vi "Autonomous Independent.vi"   [LabVIEW 2019]
doc: "This VI is called when autonomous begins, and will automatically be terminated when autonomous ends. You can carry out timed or sensor driven robot movement independently without needing to return to the caller."
uses:
  <vilib>/Rock Robotics/WPI/ThirdParty/Phoenix-LabVIEW/Motor Controller/Controls/CTRE_Phoenix_MotorControl_ControlMode.ctl
  <vilib>/Rock Robotics/WPI/Solenoid/WPI_SolenoidValue.ctl
  <vilib>/Rock Robotics/Network Tables/NT Read String.vi
  <vilib>/Rock Robotics/WPI/Utilities/WPI_GetSetVariantRefNum.vi
  <vilib>/Rock Robotics/Network Tables/NT Write Number.vi
  <vilib>/Rock Robotics/WPI/Solenoid/WPI_SolenoidSetEnum.vi
  <vilib>/Rock Robotics/Network Tables/NT Read Number.vi
  <vilib>/addons/control/pid/pid.llb/PID (DBL).vi
  <vilib>/addons/control/pid/NI_PID_pid.lvlib
  <vilib>/Rock Robotics/Network Tables/NT Write Numeric Array.vi
panel:
  # "Be sure to right-click and choose Data Operations>>Make Current Value default if you want to save the array values with the VI"
types:
  T1 = typedef "WPI_JoystickDevRef.ctl" = cluster{"Device":T2}
  T2 = typedef "WPI_JoystickDeviceEnum.ctl" = enum16{"USB 0", "USB 1", "USB 2", "USB 3", "USB 4", "USB 5"}
  T3 = typedef "WPI_MotorControlDeviceRef.ctl" = cluster{"DeviceStatus":errorcluster, "Type":T4, "PWM":cluster{"PWM Channel":T5, "DeadBand":T6}, "CAN":cluster{"Device Number":u8, "SetOutput VI Ref":variant, "GetOutput VI Ref":variant, "Enable VI Ref":variant, "Disable VI Ref":variant, "Data":variant}, "Invert":bool, "DIO PWM":cluster{"PWM \"Enable\" Channel":T5, "DIOChannel":T7, "PWM Rate":dbl}}
  T4 = typedef "WPI_MotorControlType.ctl" = enum16{"PWM", "CAN", "DIO PWM"}
  T5 = typedef "FPGA_DIOPWMChannel.ctl" = enum8{"PWM 0", "PWM 1", "PWM 2", "PWM 3", "PWM 4", "PWM 5", "PWM 6", "PWM 7", "PWM 8", "PWM 9", "PWM MXP 0", "PWM MXP 1", "PWM MXP 2", "PWM MXP 3", "PWM MXP 4", "PWM MXP 5", "PWM MXP 6", "PWM MXP 7", "PWM MXP 8", "PWM MXP 9", "Invalid"}
  T6 = typedef "WPI_PWMDeadband.ctl" = cluster{"Name":string, "maxPositivePwm":i32, "minPositivePwm":i32, "centerPwm":i32, "maxNegativePwm":i32, "minNegativePwm":i32, "angularRange":u16}
  T7 = typedef "FPGA_DIOChannel.ctl" = enum8{"DIO 0", "DIO 1", "DIO 2", "DIO 3", "DIO 4", "DIO 5", "DIO 6", "DIO 7", "DIO 8", "DIO 9", "DIO MXP 0", "DIO MXP 1", "DIO MXP 2", "DIO MXP 3", "DIO MXP 4", "DIO MXP 5", "DIO MXP 6", "DIO MXP 7", "DIO MXP 8", "DIO MXP 9", "DIO MXP 10", "DIO MXP 11", "DIO MXP 12", "DIO MXP 13", "DIO MXP 14", "DIO MXP 15", "SPI Port CS1", "SPI Port CS2", "SPI Port CS3", "SPI Port MISO", "SPI Port MOSI", "Invalid"}
  T8 = typedef "WPI_RobotDriveDevRef.ctl" = cluster{"DevStatus":errorcluster, "Motors[]":T3[], "Square Inputs":bool, "Max Output":dbl}
  T9 = typedef "WPI_GyroDevRef.ctl" = cluster{"DevStatus":errorcluster, "Analog Channel":T10, "Gain (VoltsPerDegree/Second)":dbl, "Gyro Type":enum16{"Analog", "XRS450"}, "Handle":i32, "SPI Bus":T11, "Device Found":bool, "Sample Rate":dbl, "Calibrate On Open":bool, "Offset":dbl}
  T10 = typedef "FPGA_AIChannel.ctl" = enum8{"AI 0", "AI 1", "AI 2", "AI 3", "AI MXP 0", "AI MXP 1", "AI MXP 2", "AI MXP 3", "Invalid"}
  T11 = typedef "spi_bus.ctl" = enum16{"SPI On-Board, CS0", "SPI On-Board, CS1", "SPI On-Board, CS2", "SPI On-Board, CS3", "SPI MXP", "Invalid"}
  T12 = typedef "WPI_SolenoidDevRef.ctl" = cluster{"DevStatus":errorcluster, "Pneumatics Control Module":u8, "Forward Solenoid Channel":T13, "Reverse Solenoid Channel":T13}
  T13 = typedef "WPI_SolenoidChannel.ctl" = enum8{"Solenoid 0", "Solenoid 1", "Solenoid 2", "Solenoid 3", "Solenoid 4", "Solenoid 5", "Solenoid 6", "Solenoid 7", "Invalid"}
  T14 = typedef "WPI_SolenoidValue.ctl" = enum16{"Off", "On", "Forward", "Reverse"}
  T15 = cluster{"proportional gain (Kc)":dbl, "integral time (Ti, min)":dbl, "derivative time (Td, min)":dbl}
  T16 = typedef "CTRE_Phoenix_MotorControl_ControlMode.ctl" = u16
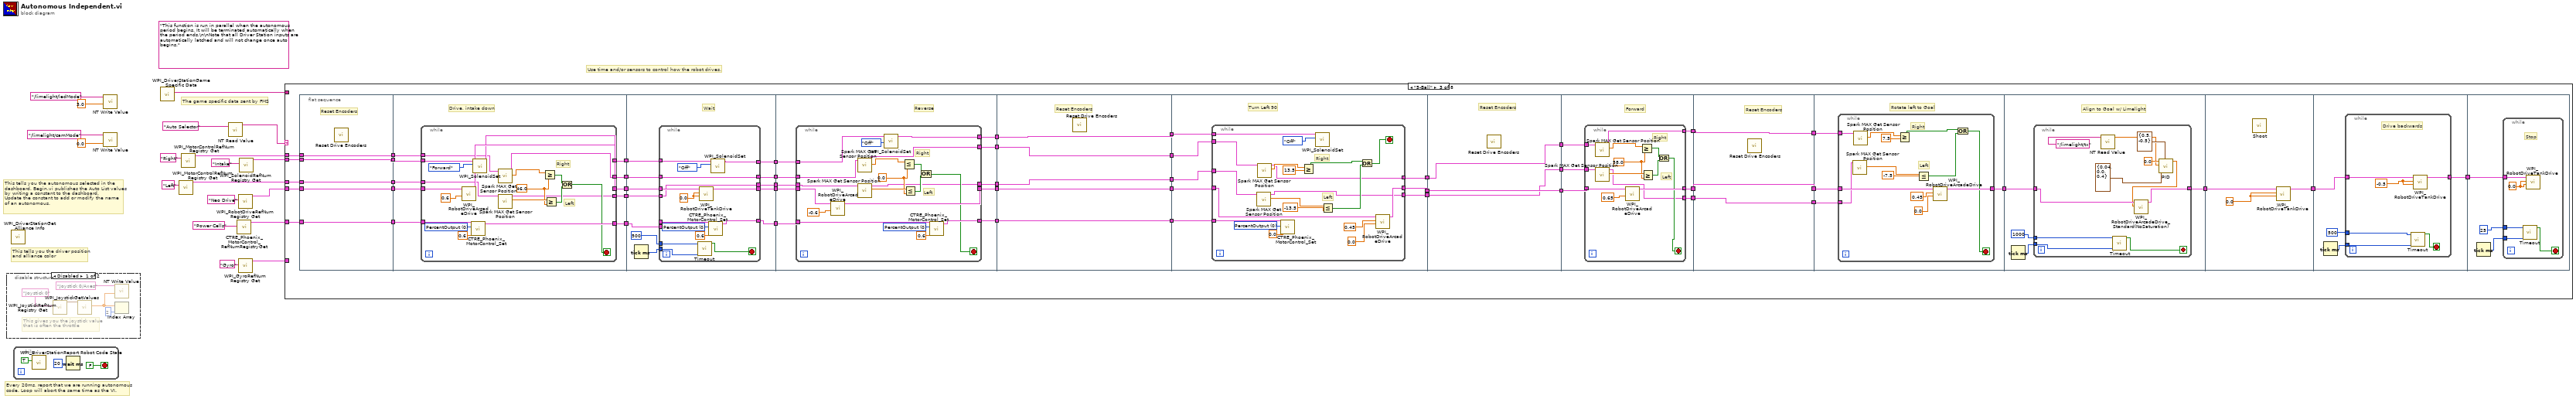
[diagram p0: block diagram]
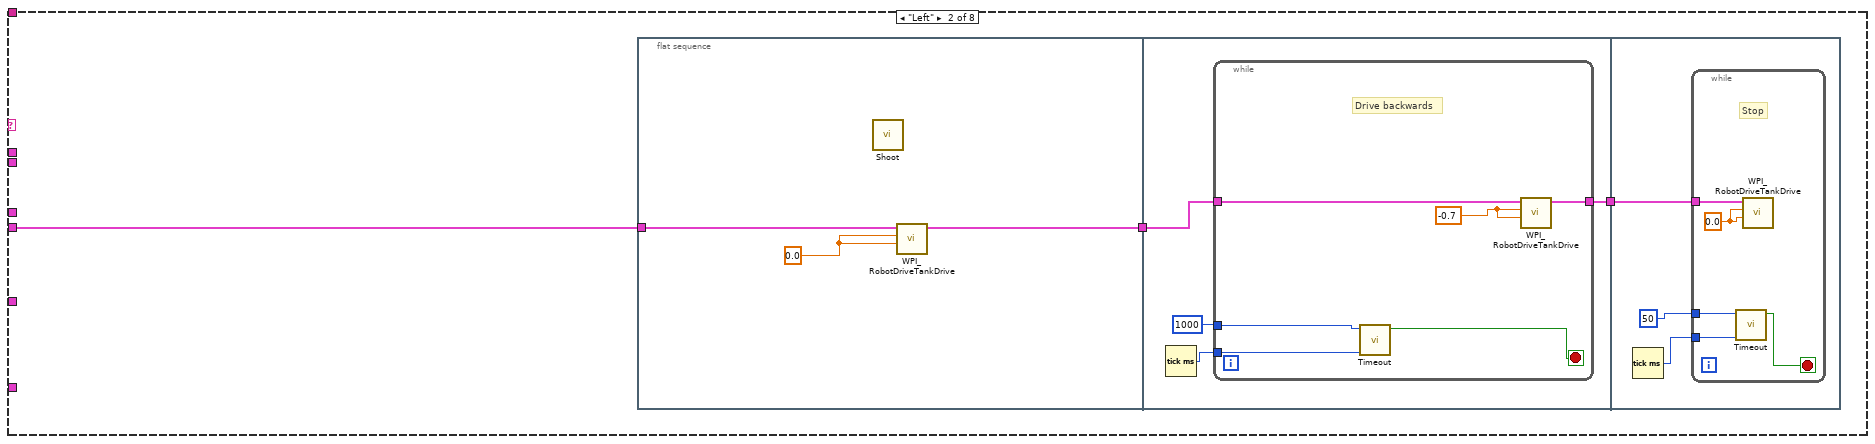
[diagram p4: hidden frame]
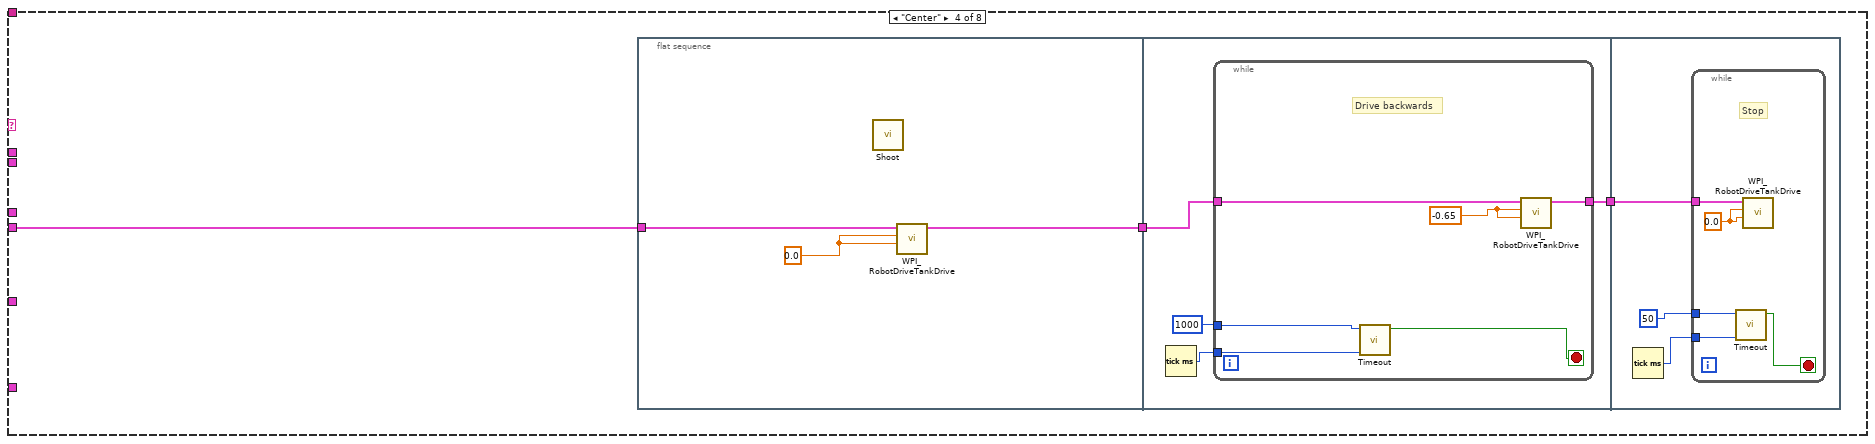
[diagram p5: hidden frame]
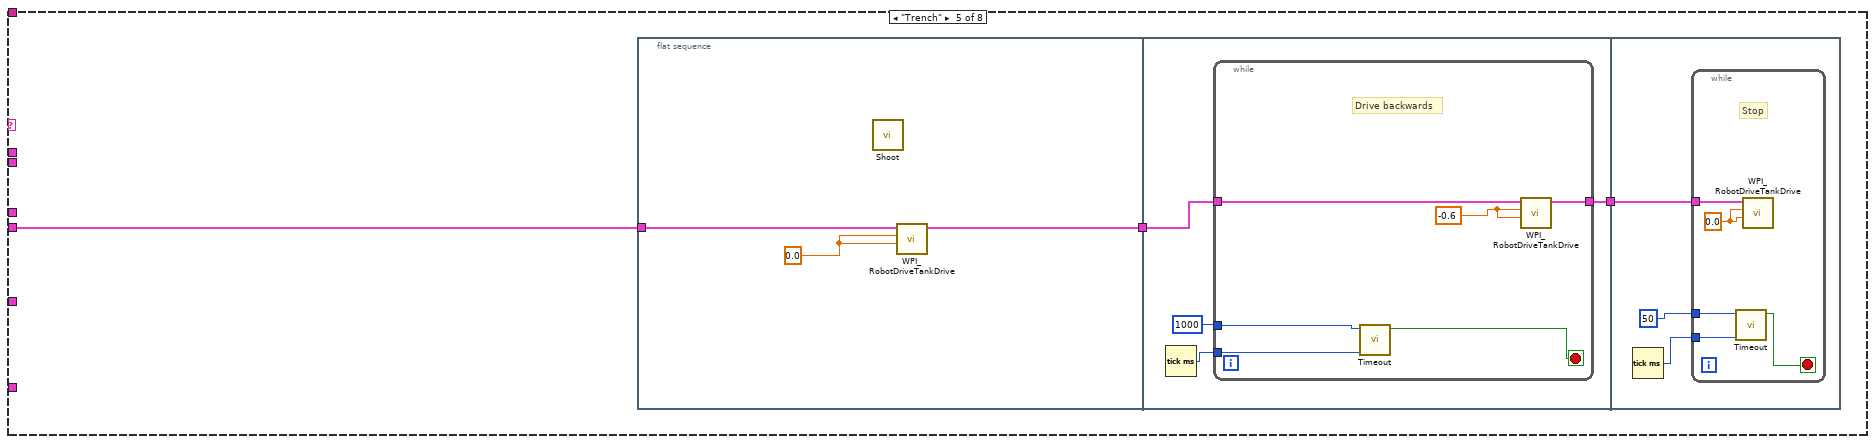
[diagram p6: hidden frame]
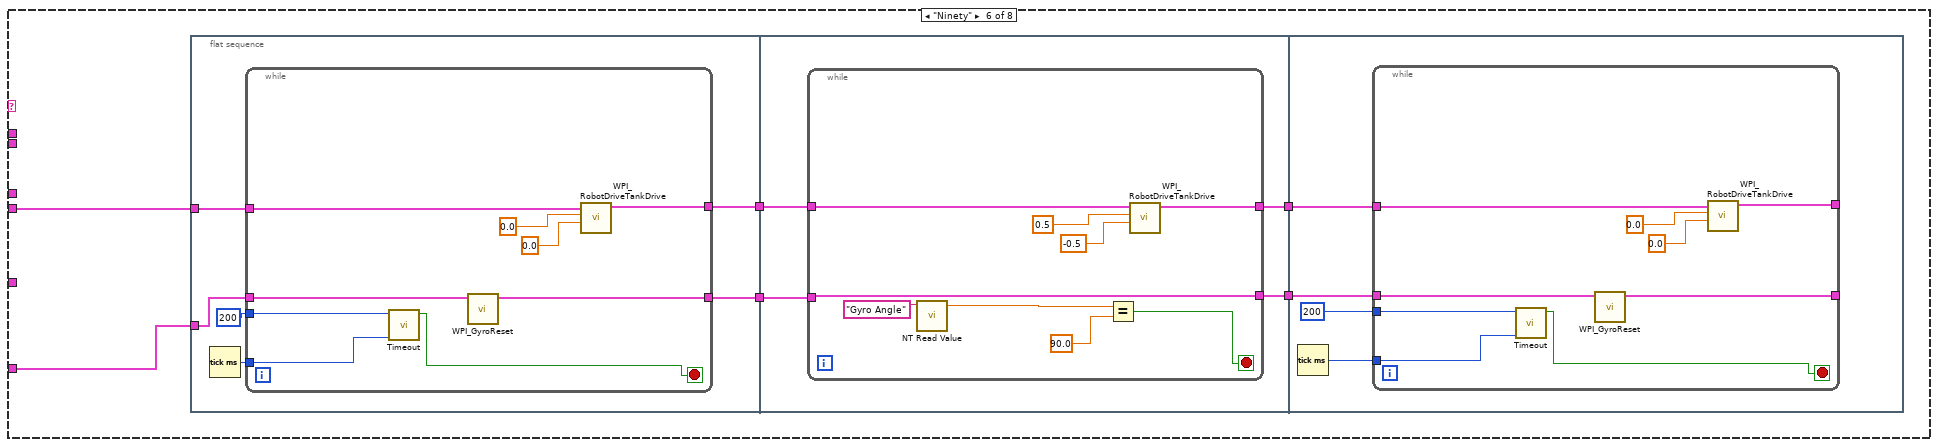
[diagram p7: hidden frame]
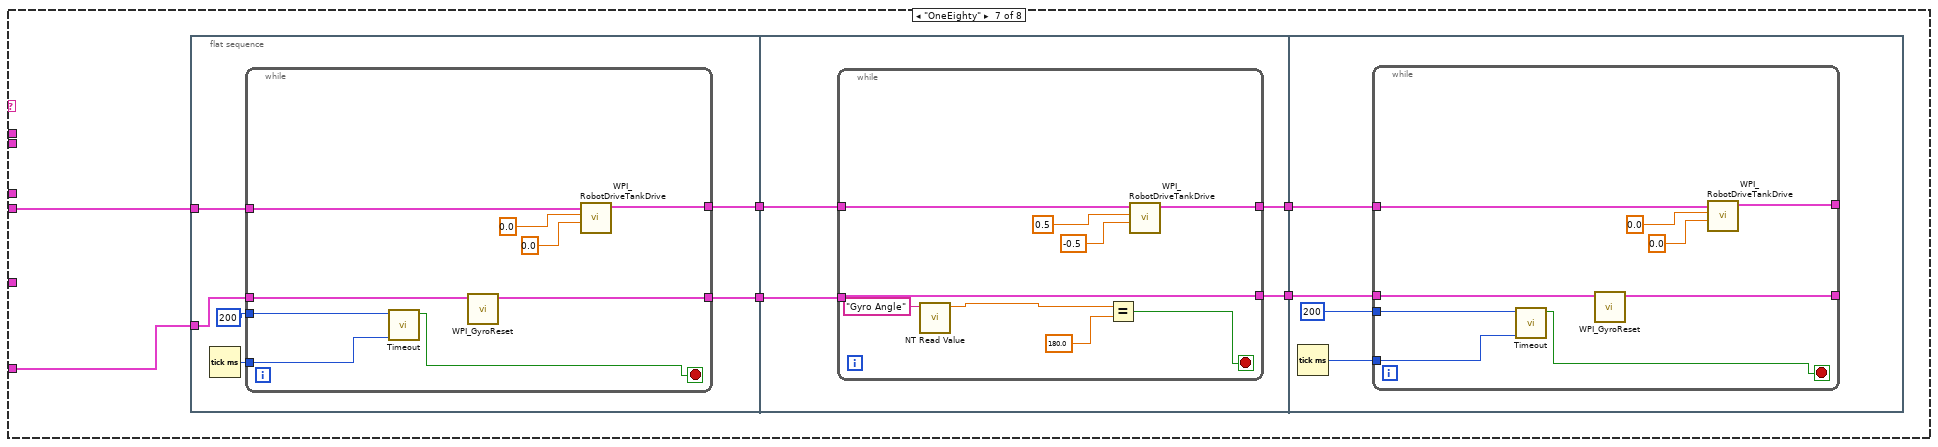
[diagram p8: hidden frame]
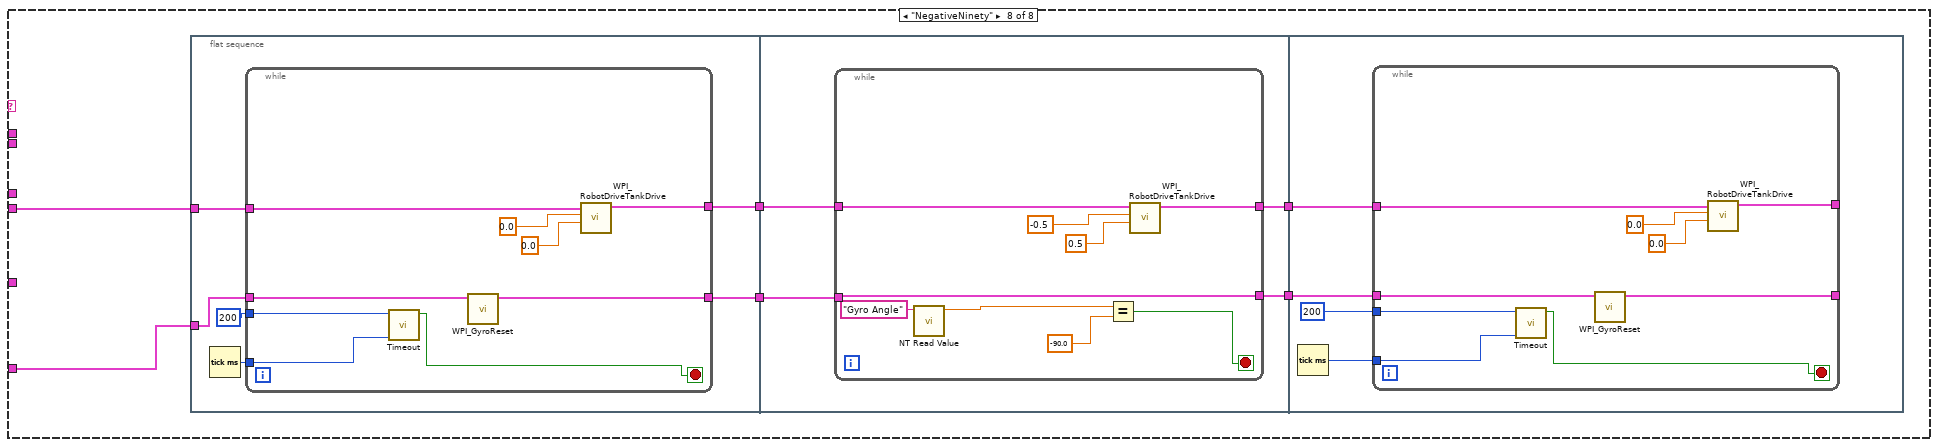
[diagram p9: hidden frame]
diagram:
  (unwired) "This function is run in parallel when the autonomous period begins. It will be terminated automatically when the period ends.\n\nNote that all Driver Station inputs are automatically latched and will not change once auto begins."
  # "The game specific data sent by FMS"
  # "This tells you the autonomous selected in the \ndashboard. Begin.vi publishes the Auto List values\nby writing a constant to the dashboard.\nUpdate the constant to add or modify the name\nof an autonomous."
  # "Every 20ms, report that we are running autonomous\ncode. Loop will abort the same time as the VI."
  # "Use time and/or sensors to control how the robot drives."
  # "This tells you the driver position\nand alliance color"
  n1 = disable-structure shown="Disabled" {
    frame Disabled {
      # "This gives you the joystick value\nthat is often the throttle"
      n2 = call <vilib>:"WPI_JoystickRefNum Registry Get.vi"("refnum name"="Joystick 0") -> ("JoystickDevRef"=w23:T1)  [unwired: 1 in, 9 out]
      n3 = call <vilib>:"WPI_JoystickGetValues.vi"("JoystickDevRef"=w23) -> ("Axes"=w21:dbl[])  [unwired: 6 in, 4 out]
      n4 = call-poly <vilib>:"NT Write Value.vi"("Numeric Array"=w21, "Name"="Joystick 0/Axes") -> ()  [unwired: 9 in, 1 out]
      n5 = Index Array(array=w21, index=2) -> ()  [unwired: 1 out]
    }
    frame Enabled {
    }
  }
  n6 = call <vilib>:"WPI_DriverStationGet Alliance Info.vi"() -> ()  [unwired: 12 out]
  n7 = while {
    stop <- FALSE stop-if-true
    n8 = call <vilib>:"WPI_DriverStationReport Robot Code State.vi"("Autonomous"=TRUE) -> ()  [unwired: 10 in, 1 out]
    n9 = Wait (ms)(milliseconds to wait=u32 20) -> ()  [unwired: 1 out]
  }
  n10 = call-poly <vilib>:"NT Write Value.vi"("Numeric"=3.0, "Name"="/limelight/ledMode") -> ()  [unwired: 9 in, 1 out]
  n11 = call-poly <vilib>:"NT Write Value.vi"("Numeric"=0.0, "Name"="/limelight/camMode") -> ()  [unwired: 9 in, 1 out]
  n12 = call <vilib>:"WPI_DriverStationGame Specific Data.vi"() -> ("Game Specific Data"=w18:string)  [unwired: 11 in]
  n13 = call <vilib>:"WPI_MotorControlRefNum Registry Get.vi"("refnum name"="Left") -> ("MotorControlDevRef"=w5:T3)  [unwired: 9 in, 1 out]
  n14 = call <vilib>:"WPI_MotorControlRefNum Registry Get.vi"("refnum name"="Right") -> ("MotorControlDevRef"=w4:T3)  [unwired: 9 in, 1 out]
  n15 = call-poly <vilib>:"NT Read Value.vi"("Name"="Auto Selector") -> ("String"=w3:string)  [unwired: 9 in, 1 out]
  n16 = call <vilib>:"CTRE_Phoenix_MotorControl_RefNumRegistryGet.vi"("refnum name"="Power Cells") -> ("PhoenixMotorControlDevRef"=w12:T3)  [unwired: 9 in, 1 out]
  n17 = call <vilib>:"WPI_RobotDriveRefNum Registry Get.vi"("refnum name"="Neo Drive") -> ("RobotDriveDevRef"=w16:T8)  [unwired: 9 in, 1 out]
  n18 = call <vilib>:"WPI_GyroRefNum Registry Get.vi"("refnum name"="Gyro") -> ("GyroDevRef"=w1:T9)  [unwired: 9 in, 1 out]
  n19 = call <vilib>:"WPI_SolenoidRefNum Registry Get.vi"("refnum name"="Intake") -> ("SolenoidDevRef"=w13:T12)  [unwired: 9 in, 1 out]
  n20 = case shown="\"5-Ball\"" w3 {
    tunnel: w18 -> [_ _ _ _ _ _ _ _]
    tunnel: w16 -> [_ w30 w97 w303 w327 w354 w401 w448]
    tunnel: w13 -> [_ _ w94 _ _ _ _ _]
    tunnel: w12 -> [_ _ w93 _ _ _ _ _]
    tunnel: w5 -> [_ _ w78 _ _ _ _ _]
    tunnel: w4 -> [_ _ w79 _ _ _ _ _]
    tunnel: w1 -> [_ _ _ _ _ w353 w400 w447]
    frame Default {
      # "You can put your main auto here, or you can right-click on the case and make any\nother frame be the default case."
      # "This is the frame that will execute if no selection is made, or if it is not recognized"
    }
    frame "Left" {
      n21 = flat-sequence {
        tunnel: w30 -> [w33]
        tunnel: [w32] -> w29
        tunnel: w29 -> [w35]
        tunnel: [w34] -> w28
        tunnel: w28 -> [w44]
        frame #0 {
          w31 = 0.0 ("Left axis value")
          n22 = call "Shoot.vi"() -> ()  [unwired: 12 in]
          n23 = call <vilib>:"WPI_RobotDriveTankDrive.vi"("Right axis value"=w31, "Left axis value"=w31, "RobotDriveDevRef"=w33) -> ("RobotDriveDevRef"=w32:T8)  [unwired: 6 in, 2 out]
        }
        frame #1 {
          n24 = Tick Count (ms)() -> (millisecond timer value=w37:u32)
          n25 = while {
            tunnel: w35 -> [w43]
            tunnel: w37 -> [w41]
            tunnel: 1000 -> [w40]
            tunnel: [w38] -> w34
            stop <- w39 stop-if-true
            w42 = -0.7 ("Left axis value")
            # "Drive backwards"
            n26 = call "Timeout.vi"("Start Time In"=w41, "Limit In"=w40) -> ("Timeout"=w39:bool)  [unwired: 8 in, 1 out]
            n27 = call <vilib>:"WPI_RobotDriveTankDrive.vi"("Right axis value"=w42, "Left axis value"=w42, "RobotDriveDevRef"=w43) -> ("RobotDriveDevRef"=w38:T8)  [unwired: 6 in, 2 out]
          }
        }
        frame #2 {
          n28 = Tick Count (ms)() -> (millisecond timer value=w46:u32)
          n29 = while {
            tunnel: w46 -> [w51]
            tunnel: 50 -> [w50]
            tunnel: w44 -> [w48]
            stop <- w49 stop-if-true
            w47 = 0.0 ("Left axis value")
            # "Stop"
            n30 = call "Timeout.vi"("Start Time In"=w51, "Limit In"=w50) -> ("Timeout"=w49:bool)  [unwired: 8 in, 1 out]
            n31 = call <vilib>:"WPI_RobotDriveTankDrive.vi"("Right axis value"=w47, "Left axis value"=w47, "RobotDriveDevRef"=w48) -> ()  [unwired: 6 in, 3 out]
          }
        }
      }
    }
    frame "5-Ball" {
      n32 = flat-sequence {
        tunnel: w78 -> [w100]
        tunnel: w79 -> [w98]
        tunnel: w93 -> [w102]
        tunnel: w94 -> [w99]
        tunnel: w97 -> [w101]
        tunnel: [w102] -> w71
        tunnel: [w101] -> w58
        tunnel: [w100] -> w57
        tunnel: [w99] -> w56
        tunnel: [w98] -> w55
        tunnel: [w110] -> w90
        tunnel: [w108] -> w88
        tunnel: [w107] -> w87
        tunnel: [w104] -> w77
        tunnel: [w103] -> w76
        tunnel: w71 -> [w112]
        tunnel: w58 -> [w111]
        tunnel: w57 -> [w105]
        tunnel: w56 -> [w109]
        tunnel: w55 -> [w106]
        tunnel: w90 -> [w140]
        tunnel: [w143] -> w89
        tunnel: w88 -> [w144]
        tunnel: w87 -> [w142]
        tunnel: [w141] -> w86
        tunnel: [w137] -> w81
        tunnel: w77 -> [w136]
        tunnel: w76 -> [w135]
        tunnel: [w134] -> w75
        tunnel: [w133] -> w74
        tunnel: [w168] -> w85
        tunnel: w89 -> [w169]
        tunnel: w86 -> [w167]
        tunnel: [w166] -> w83
        tunnel: w81 -> [w165]
        tunnel: [w164] -> w80
        tunnel: w75 -> [w163]
        tunnel: w74 -> [w162]
        tunnel: [w161] -> w73
        tunnel: [w160] -> w72
        tunnel: w85 -> [w194]
        tunnel: [w194] -> w84
        tunnel: w83 -> [w193]
        tunnel: [w193] -> w82
        tunnel: w80 -> [w190]
        tunnel: w73 -> [w191]
        tunnel: w72 -> [w192]
        tunnel: [w192] -> w54
        tunnel: [w191] -> w53
        tunnel: [w190] -> w52
        tunnel: w84 -> [w202]
        tunnel: [w201] -> w70
        tunnel: w82 -> [w200]
        tunnel: [w196] -> w68
        tunnel: [w195] -> w67
        tunnel: w54 -> [w199]
        tunnel: w53 -> [w198]
        tunnel: w52 -> [w197]
        tunnel: w70 -> [w225]
        tunnel: [w225] -> w69
        tunnel: w68 -> [w224]
        tunnel: w67 -> [w223]
        tunnel: [w224] -> w66
        tunnel: [w223] -> w65
        tunnel: w69 -> [w231]
        tunnel: [w230] -> w64
        tunnel: w66 -> [w229]
        tunnel: w65 -> [w228]
        tunnel: [w227] -> w62
        tunnel: [w226] -> w61
        tunnel: w64 -> [w247]
        tunnel: [w247] -> w63
        tunnel: w62 -> [w246]
        tunnel: w61 -> [w245]
        tunnel: [w246] -> w60
        tunnel: [w245] -> w59
        tunnel: w63 -> [w251]
        tunnel: [w250] -> w92
        tunnel: w60 -> [w249]
        tunnel: w59 -> [w248]
        tunnel: w92 -> [w268]
        tunnel: [w267] -> w91
        tunnel: [w281] -> w96
        tunnel: w91 -> [w282]
        tunnel: w96 -> [w284]
        tunnel: [w283] -> w95
        tunnel: w95 -> [w293]
        frame #0 {
          # "Reset Encoders"
          n33 = call "Reset Drive Encoders.vi"() -> ()  [unwired: 12 in]
        }
        frame #1 {
          # "Drive, intake down"
          n34 = while {
            tunnel: w112 -> [w132]
            tunnel: w111 -> [w129]
            tunnel: [w128] -> w110
            tunnel: w109 -> [w126]
            tunnel: [w124] -> w108
            tunnel: [w123] -> w107
            tunnel: w106 -> [w116]
            tunnel: w105 -> [w115]
            tunnel: [w114] -> w104
            tunnel: [w113] -> w103
            stop <- w117 stop-if-true
            w120 = 46.0 ("y")
            w131 = T16 0 items=["PercentOutput"=0, "Position"=1, "Velocity"=2, "Current"=3, "Follower"=5, "MotionProfile"=6, "MotionMagic"=7, "MotionProfileArc"=10, "Disabled"=15] ("Control Mode")
            # "Left"
            # "Right"
            n35 = call-poly <vilib>:"WPI_RobotDriveArcadeDrive.vi"("Y axis value"=0.6 ("Left axis value"), "RobotDriveDevRef"=w129) -> ("RobotDriveDevRef"=w128:T8)  [unwired: 7 in, 2 out]
            n36 = call <vilib>:"CTRE_Phoenix_MotorControl_Set.vi"("Output"=0.6, "Control Mode"=w131, "PhoenixMotorControlDevRef"=w132) -> ("PhoenixMotorControlDevRef"=w123:T3)  [unwired: 7 in, 1 out]
            n37 = call-poly <vilib>:"WPI_SolenoidSet.vi"("Value"=WPI_SolenoidValue."Forward", "SolenoidDevRef"=w126) -> ("SolenoidDevRef"=w124:T12)  [unwired: 8 in, 1 out]
            n38 = call <vilib>:"Spark MAX Get Sensor Position.vi"("MotorControlDevRef in"=w116) -> ("Sensor Position"=w122:dbl, "MotorControlDevRef out"=w114:T3)  [unwired: 7 in, 2 out]
            n39 = call <vilib>:"Spark MAX Get Sensor Position.vi"("MotorControlDevRef in"=w115) -> ("Sensor Position"=w121:dbl, "MotorControlDevRef out"=w113:T3)  [unwired: 7 in, 2 out]
            n40 = Greater Or Equal?(x=w122, y=w120) -> (x >= y?=w118:bool)
            n41 = Greater Or Equal?(x=w121, y=w120) -> (x >= y?=w119:bool)
            n42 = Or(x=w118, y=w119) -> (x .or. y?=w117:bool)
          }
        }
        frame #2 {
          # "Wait"
          n43 = Tick Count (ms)() -> (millisecond timer value=w139:u32)
          n44 = while {
            tunnel: [w148] -> _
            tunnel: 500 -> [w156]
            tunnel: w139 -> [w155]
            tunnel: w140 -> [w154]
            tunnel: [w153] -> w143
            tunnel: w144 -> [w151]
            tunnel: [w149] -> w141
            tunnel: w142 -> [w148]
            tunnel: [w147] -> w137
            tunnel: w136 -> [w146]
            tunnel: w135 -> [w145]
            tunnel: [w146] -> w134
            tunnel: [w145] -> w133
            stop <- w157 stop-if-true
            w152 = 0.0 ("Left axis value")
            w159 = T16 0 items=["PercentOutput"=0, "Position"=1, "Velocity"=2, "Current"=3, "Follower"=5, "MotionProfile"=6, "MotionMagic"=7, "MotionProfileArc"=10, "Disabled"=15] ("Control Mode")
            n45 = call "Timeout.vi"("Start Time In"=w155, "Limit In"=w156) -> ("Timeout"=w157:bool)  [unwired: 8 in, 1 out]
            n46 = call <vilib>:"WPI_RobotDriveTankDrive.vi"("Right axis value"=w152, "Left axis value"=w152, "RobotDriveDevRef"=w154) -> ("RobotDriveDevRef"=w153:T8)  [unwired: 6 in, 2 out]
            n47 = call <vilib>:"CTRE_Phoenix_MotorControl_Set.vi"("Output"=0.6, "Control Mode"=w159, "PhoenixMotorControlDevRef"=w148) -> ("PhoenixMotorControlDevRef"=w149:T3)  [unwired: 7 in, 1 out]
            n48 = call-poly <vilib>:"WPI_SolenoidSet.vi"("Value"=WPI_SolenoidValue."Off", "SolenoidDevRef"=w151) -> ("SolenoidDevRef"=w147:T12)  [unwired: 8 in, 1 out]
          }
        }
        frame #3 {
          # "Reverse"
          n49 = while {
            tunnel: w167 -> [w189]
            tunnel: w169 -> [w186]
            tunnel: [w185] -> w168
            tunnel: [w183] -> w166
            tunnel: w165 -> [w181]
            tunnel: [w180] -> w164
            tunnel: w163 -> [w174]
            tunnel: w162 -> [w173]
            tunnel: [w171] -> w161
            tunnel: [w170] -> w160
            stop <- w172 stop-if-true
            w177 = 0.0 ("y")
            w188 = T16 0 items=["PercentOutput"=0, "Position"=1, "Velocity"=2, "Current"=3, "Follower"=5, "MotionProfile"=6, "MotionMagic"=7, "MotionProfileArc"=10, "Disabled"=15] ("Control Mode")
            # "Left"
            # "Right"
            n50 = call-poly <vilib>:"WPI_RobotDriveArcadeDrive.vi"("Y axis value"=-0.6 ("Left axis value"), "RobotDriveDevRef"=w186) -> ("RobotDriveDevRef"=w185:T8)  [unwired: 7 in, 2 out]
            n51 = call <vilib>:"Spark MAX Get Sensor Position.vi"("MotorControlDevRef in"=w174) -> ("Sensor Position"=w179:dbl, "MotorControlDevRef out"=w171:T3)  [unwired: 7 in, 2 out]
            n52 = call <vilib>:"Spark MAX Get Sensor Position.vi"("MotorControlDevRef in"=w173) -> ("Sensor Position"=w178:dbl, "MotorControlDevRef out"=w170:T3)  [unwired: 7 in, 2 out]
            n53 = call-poly <vilib>:"WPI_SolenoidSet.vi"("Value"=WPI_SolenoidValue."Off", "SolenoidDevRef"=w181) -> ("SolenoidDevRef"=w180:T12)  [unwired: 8 in, 1 out]
            n54 = Less Or Equal?(x=w179, y=w177) -> (x <= y?=w175:bool)
            n55 = Less Or Equal?(x=w178, y=w177) -> (x <= y?=w176:bool)
            n56 = Or(x=w175, y=w176) -> (x .or. y?=w172:bool)
            n57 = call <vilib>:"CTRE_Phoenix_MotorControl_Set.vi"("Output"=0.6, "Control Mode"=w188, "PhoenixMotorControlDevRef"=w189) -> ("PhoenixMotorControlDevRef"=w183:T3)  [unwired: 7 in, 1 out]
          }
        }
        frame #4 {
          # "Reset Encoders"
          n58 = call "Reset Drive Encoders.vi"() -> ()  [unwired: 12 in]
        }
        frame #5 {
          # "Turn Left 90"
          n59 = while {
            tunnel: w202 -> [w222]
            tunnel: [w221] -> w201
            tunnel: w200 -> [w216]
            tunnel: w198 -> [w215]
            tunnel: w199 -> [w214]
            tunnel: w197 -> [w205]
            tunnel: [w204] -> w196
            tunnel: [w203] -> w195
            stop <- w213 stop-if-true
            w218 = T16 0 items=["PercentOutput"=0, "Position"=1, "Velocity"=2, "Current"=3, "Follower"=5, "MotionProfile"=6, "MotionMagic"=7, "MotionProfileArc"=10, "Disabled"=15] ("Control Mode")
            # "Left"
            # "Right"
            n60 = call <vilib>:"Spark MAX Get Sensor Position.vi"("MotorControlDevRef in"=w214) -> ("Sensor Position"=w208:dbl, "MotorControlDevRef out"=w203:T3)  [unwired: 7 in, 2 out]
            n61 = call <vilib>:"Spark MAX Get Sensor Position.vi"("MotorControlDevRef in"=w215) -> ("Sensor Position"=w212:dbl, "MotorControlDevRef out"=w204:T3)  [unwired: 7 in, 2 out]
            n62 = call <vilib>:"CTRE_Phoenix_MotorControl_Set.vi"("Output"=0.0, "Control Mode"=w218, "PhoenixMotorControlDevRef"=w216) -> ()  [unwired: 7 in, 2 out]
            n63 = Greater Or Equal?(x=w212, y=13.5) -> (x >= y?=w210:bool)
            n64 = call-poly <vilib>:"WPI_SolenoidSet.vi"("Value"=WPI_SolenoidValue."Off", "SolenoidDevRef"=w205) -> ()  [unwired: 8 in, 2 out]
            n65 = Less Or Equal?(x=w208, y=-13.5) -> (x <= y?=w207:bool)
            n66 = Or(x=w210, y=w207) -> (x .or. y?=w213:bool)
            n67 = call-poly <vilib>:"WPI_RobotDriveArcadeDrive.vi"("Y axis value"=0.0 ("Left axis value"), "X axis value"=0.45 ("Left axis value"), "RobotDriveDevRef"=w222) -> ("RobotDriveDevRef"=w221:T8)  [unwired: 6 in, 2 out]
          }
        }
        frame #6 {
          # "Reset Encoders"
          n68 = call "Reset Drive Encoders.vi"() -> ()  [unwired: 12 in]
        }
        frame #7 {
          # "Forward"
          n69 = while {
            tunnel: w231 -> [w244]
            tunnel: [w243] -> w230
            tunnel: w229 -> [w235]
            tunnel: w228 -> [w234]
            tunnel: [w233] -> w227
            tunnel: [w232] -> w226
            stop <- w236 stop-if-true
            w239 = 58.0 ("y")
            # "Left"
            # "Right"
            n70 = call <vilib>:"Spark MAX Get Sensor Position.vi"("MotorControlDevRef in"=w235) -> ("Sensor Position"=w241:dbl, "MotorControlDevRef out"=w233:T3)  [unwired: 7 in, 2 out]
            n71 = call <vilib>:"Spark MAX Get Sensor Position.vi"("MotorControlDevRef in"=w234) -> ("Sensor Position"=w240:dbl, "MotorControlDevRef out"=w232:T3)  [unwired: 7 in, 2 out]
            n72 = call-poly <vilib>:"WPI_RobotDriveArcadeDrive.vi"("Y axis value"=0.65 ("Left axis value"), "RobotDriveDevRef"=w244) -> ("RobotDriveDevRef"=w243:T8)  [unwired: 7 in, 2 out]
            n73 = Greater Or Equal?(x=w241, y=w239) -> (x >= y?=w237:bool)
            n74 = Greater Or Equal?(x=w240, y=w239) -> (x >= y?=w238:bool)
            n75 = Or(x=w237, y=w238) -> (x .or. y?=w236:bool)
          }
        }
        frame #8 {
          # "Reset Encoders"
          n76 = call "Reset Drive Encoders.vi"() -> ()  [unwired: 12 in]
        }
        frame #9 {
          # "Rotate left to Goal"
          n77 = while {
            tunnel: w251 -> [w264]
            tunnel: [w263] -> w250
            tunnel: w249 -> [w253]
            tunnel: w248 -> [w252]
            stop <- w254 stop-if-true
            # "Left"
            # "Right"
            n78 = call <vilib>:"Spark MAX Get Sensor Position.vi"("MotorControlDevRef in"=w252) -> ("Sensor Position"=w256:dbl)  [unwired: 7 in, 3 out]
            n79 = call <vilib>:"Spark MAX Get Sensor Position.vi"("MotorControlDevRef in"=w253) -> ("Sensor Position"=w260:dbl)  [unwired: 7 in, 3 out]
            n80 = Greater Or Equal?(x=w260, y=7.5) -> (x >= y?=w258:bool)
            n81 = Less Or Equal?(x=w256, y=-7.5) -> (x <= y?=w255:bool)
            n82 = call-poly <vilib>:"WPI_RobotDriveArcadeDrive.vi"("Y axis value"=0.0 ("Left axis value"), "X axis value"=0.45 ("Left axis value"), "RobotDriveDevRef"=w264) -> ("RobotDriveDevRef"=w263:T8)  [unwired: 6 in, 2 out]
            n83 = Or(x=w258, y=w255) -> (x .or. y?=w254:bool)
          }
        }
        frame #10 {
          # "Align to Goal w/ Limelight"
          n84 = Tick Count (ms)() -> (millisecond timer value=w265:u32)
          n85 = while {
            tunnel: w268 -> [w271]
            tunnel: [w270] -> w267
            tunnel: 1000 -> [w279]
            tunnel: w265 -> [w278]
            stop <- w277 stop-if-true
            n86 = call-poly <vilib>:"NT Read Value.vi"("Name"="/limelight/tx") -> ("Numeric"=w274:dbl)  [unwired: 9 in, 1 out]
            n87 = call "Timeout.vi"("Start Time In"=w278, "Limit In"=w279) -> ("Timeout"=w277:bool)  [unwired: 8 in, 1 out]
            n88 = call-poly <vilib>:"PID.vi"("output range"=cluster{"output high":dbl, "output low":dbl} {"output high"=0.5, "output low"=-0.5}, "PID gains"=T15 {"proportional gain (Kc)"=0.04, "integral time (Ti, min)"=0.0, "derivative time (Td, min)"=0.4}, "process variable"=w274, "setpoint"=0.0) -> ("output"=w269:dbl)  [unwired: 6 in, 1 out]
            n89 = call <vilib>:"WPI_RobotDriveArcadeDrive_Standard(NoSaturation).vi"("X axis value"=w269, "RobotDriveDevRef"=w271) -> ("RobotDriveDevRef"=w270:T8)  [unwired: 2 in, 7 out]
          }
        }
        frame #11 {
          w280 = 0.0 ("Left axis value")
          n90 = call "Shoot.vi"() -> ()  [unwired: 12 in]
          n91 = call <vilib>:"WPI_RobotDriveTankDrive.vi"("Right axis value"=w280, "Left axis value"=w280, "RobotDriveDevRef"=w282) -> ("RobotDriveDevRef"=w281:T8)  [unwired: 6 in, 2 out]
        }
        frame #12 {
          n92 = Tick Count (ms)() -> (millisecond timer value=w286:u32)
          n93 = while {
            tunnel: w284 -> [w292]
            tunnel: w286 -> [w290]
            tunnel: 500 -> [w289]
            tunnel: [w287] -> w283
            stop <- w288 stop-if-true
            w291 = -0.5 ("Left axis value")
            # "Drive backwards"
            n94 = call "Timeout.vi"("Start Time In"=w290, "Limit In"=w289) -> ("Timeout"=w288:bool)  [unwired: 8 in, 1 out]
            n95 = call <vilib>:"WPI_RobotDriveTankDrive.vi"("Right axis value"=w291, "Left axis value"=w291, "RobotDriveDevRef"=w292) -> ("RobotDriveDevRef"=w287:T8)  [unwired: 6 in, 2 out]
          }
        }
        frame #13 {
          n96 = Tick Count (ms)() -> (millisecond timer value=w295:u32)
          n97 = while {
            tunnel: w295 -> [w300]
            tunnel: 25 -> [w299]
            tunnel: w293 -> [w297]
            stop <- w298 stop-if-true
            w296 = 0.0 ("Left axis value")
            # "Stop"
            n98 = call "Timeout.vi"("Start Time In"=w300, "Limit In"=w299) -> ("Timeout"=w298:bool)  [unwired: 8 in, 1 out]
            n99 = call <vilib>:"WPI_RobotDriveTankDrive.vi"("Right axis value"=w296, "Left axis value"=w296, "RobotDriveDevRef"=w297) -> ()  [unwired: 6 in, 3 out]
          }
        }
      }
    }
    frame "Center" {
      n100 = flat-sequence {
        tunnel: w303 -> [w306]
        tunnel: [w305] -> w302
        tunnel: w302 -> [w308]
        tunnel: [w307] -> w301
        tunnel: w301 -> [w317]
        frame #0 {
          w304 = 0.0 ("Left axis value")
          n101 = call "Shoot.vi"() -> ()  [unwired: 12 in]
          n102 = call <vilib>:"WPI_RobotDriveTankDrive.vi"("Right axis value"=w304, "Left axis value"=w304, "RobotDriveDevRef"=w306) -> ("RobotDriveDevRef"=w305:T8)  [unwired: 6 in, 2 out]
        }
        frame #1 {
          n103 = Tick Count (ms)() -> (millisecond timer value=w310:u32)
          n104 = while {
            tunnel: w308 -> [w316]
            tunnel: w310 -> [w314]
            tunnel: 1000 -> [w313]
            tunnel: [w311] -> w307
            stop <- w312 stop-if-true
            w315 = -0.65 ("Left axis value")
            # "Drive backwards"
            n105 = call "Timeout.vi"("Start Time In"=w314, "Limit In"=w313) -> ("Timeout"=w312:bool)  [unwired: 8 in, 1 out]
            n106 = call <vilib>:"WPI_RobotDriveTankDrive.vi"("Right axis value"=w315, "Left axis value"=w315, "RobotDriveDevRef"=w316) -> ("RobotDriveDevRef"=w311:T8)  [unwired: 6 in, 2 out]
          }
        }
        frame #2 {
          n107 = Tick Count (ms)() -> (millisecond timer value=w319:u32)
          n108 = while {
            tunnel: w319 -> [w324]
            tunnel: 50 -> [w323]
            tunnel: w317 -> [w321]
            stop <- w322 stop-if-true
            w320 = 0.0 ("Left axis value")
            # "Stop"
            n109 = call "Timeout.vi"("Start Time In"=w324, "Limit In"=w323) -> ("Timeout"=w322:bool)  [unwired: 8 in, 1 out]
            n110 = call <vilib>:"WPI_RobotDriveTankDrive.vi"("Right axis value"=w320, "Left axis value"=w320, "RobotDriveDevRef"=w321) -> ()  [unwired: 6 in, 3 out]
          }
        }
      }
    }
    frame "Trench" {
      n111 = flat-sequence {
        tunnel: w327 -> [w330]
        tunnel: [w329] -> w326
        tunnel: w326 -> [w332]
        tunnel: [w331] -> w325
        tunnel: w325 -> [w341]
        frame #0 {
          w328 = 0.0 ("Left axis value")
          n112 = call "Shoot.vi"() -> ()  [unwired: 12 in]
          n113 = call <vilib>:"WPI_RobotDriveTankDrive.vi"("Right axis value"=w328, "Left axis value"=w328, "RobotDriveDevRef"=w330) -> ("RobotDriveDevRef"=w329:T8)  [unwired: 6 in, 2 out]
        }
        frame #1 {
          n114 = Tick Count (ms)() -> (millisecond timer value=w334:u32)
          n115 = while {
            tunnel: w332 -> [w340]
            tunnel: w334 -> [w338]
            tunnel: 1000 -> [w337]
            tunnel: [w335] -> w331
            stop <- w336 stop-if-true
            w339 = -0.6 ("Left axis value")
            # "Drive backwards"
            n116 = call "Timeout.vi"("Start Time In"=w338, "Limit In"=w337) -> ("Timeout"=w336:bool)  [unwired: 8 in, 1 out]
            n117 = call <vilib>:"WPI_RobotDriveTankDrive.vi"("Right axis value"=w339, "Left axis value"=w339, "RobotDriveDevRef"=w340) -> ("RobotDriveDevRef"=w335:T8)  [unwired: 6 in, 2 out]
          }
        }
        frame #2 {
          n118 = Tick Count (ms)() -> (millisecond timer value=w343:u32)
          n119 = while {
            tunnel: w343 -> [w348]
            tunnel: 50 -> [w347]
            tunnel: w341 -> [w345]
            stop <- w346 stop-if-true
            w344 = 0.0 ("Left axis value")
            # "Stop"
            n120 = call "Timeout.vi"("Start Time In"=w348, "Limit In"=w347) -> ("Timeout"=w346:bool)  [unwired: 8 in, 1 out]
            n121 = call <vilib>:"WPI_RobotDriveTankDrive.vi"("Right axis value"=w344, "Left axis value"=w344, "RobotDriveDevRef"=w345) -> ()  [unwired: 6 in, 3 out]
          }
        }
      }
    }
    frame "Ninety" {
      n122 = flat-sequence {
        tunnel: w354 -> [w360]
        tunnel: w353 -> [w359]
        tunnel: [w356] -> w352
        tunnel: [w355] -> w351
        tunnel: w352 -> [w373]
        tunnel: w351 -> [w372]
        tunnel: [w371] -> w350
        tunnel: [w370] -> w349
        tunnel: w350 -> [w384]
        tunnel: w349 -> [w383]
        frame #0 {
          n123 = Tick Count (ms)() -> (millisecond timer value=w358:u32)
          n124 = while {
            tunnel: w360 -> [w369]
            tunnel: w359 -> [w366]
            tunnel: w358 -> [w365]
            tunnel: 200 -> [w364]
            tunnel: [w362] -> w356
            tunnel: [w361] -> w355
            stop <- w363 stop-if-true
            n125 = call "Timeout.vi"("Start Time In"=w365, "Limit In"=w364) -> ("Timeout"=w363:bool)  [unwired: 8 in, 1 out]
            n126 = call <vilib>:"WPI_GyroReset.vi"("GyroDevRef"=w366) -> ("GyroDevRef"=w361:T9)  [unwired: 9 in, 1 out]
            n127 = call <vilib>:"WPI_RobotDriveTankDrive.vi"("Right axis value"=0.0, "Left axis value"=0.0, "RobotDriveDevRef"=w369) -> ("RobotDriveDevRef"=w362:T8)  [unwired: 6 in, 2 out]
          }
        }
        frame #1 {
          n128 = while {
            tunnel: w373 -> [w382]
            tunnel: w372 -> [w376]
            tunnel: [w377] -> w371
            tunnel: [w376] -> w370
            stop <- w378 stop-if-true
            n129 = call-poly <vilib>:"NT Read Value.vi"("Name"="Gyro Angle") -> ("Numeric"=w375:dbl)  [unwired: 9 in, 1 out]
            n130 = Equal?(x=w375, y=90.0) -> (x = y?=w378:bool)
            n131 = call <vilib>:"WPI_RobotDriveTankDrive.vi"("Right axis value"=-0.5, "Left axis value"=0.5, "RobotDriveDevRef"=w382) -> ("RobotDriveDevRef"=w377:T8)  [unwired: 6 in, 2 out]
          }
        }
        frame #2 {
          n132 = Tick Count (ms)() -> (millisecond timer value=w386:u32)
          n133 = while {
            tunnel: w384 -> [w395]
            tunnel: w383 -> [w392]
            tunnel: w386 -> [w391]
            tunnel: 200 -> [w390]
            tunnel: [w388] -> _
            tunnel: [w387] -> _
            stop <- w389 stop-if-true
            n134 = call "Timeout.vi"("Start Time In"=w391, "Limit In"=w390) -> ("Timeout"=w389:bool)  [unwired: 8 in, 1 out]
            n135 = call <vilib>:"WPI_GyroReset.vi"("GyroDevRef"=w392) -> ("GyroDevRef"=w387:T9)  [unwired: 9 in, 1 out]
            n136 = call <vilib>:"WPI_RobotDriveTankDrive.vi"("Right axis value"=0.0, "Left axis value"=0.0, "RobotDriveDevRef"=w395) -> ("RobotDriveDevRef"=w388:T8)  [unwired: 6 in, 2 out]
          }
        }
      }
    }
    frame "OneEighty" {
      n137 = flat-sequence {
        tunnel: w401 -> [w407]
        tunnel: w400 -> [w406]
        tunnel: [w403] -> w399
        tunnel: [w402] -> w398
        tunnel: w399 -> [w420]
        tunnel: w398 -> [w419]
        tunnel: [w418] -> w397
        tunnel: [w417] -> w396
        tunnel: w397 -> [w431]
        tunnel: w396 -> [w430]
        frame #0 {
          n138 = Tick Count (ms)() -> (millisecond timer value=w405:u32)
          n139 = while {
            tunnel: w407 -> [w416]
            tunnel: w406 -> [w413]
            tunnel: w405 -> [w412]
            tunnel: 200 -> [w411]
            tunnel: [w409] -> w403
            tunnel: [w408] -> w402
            stop <- w410 stop-if-true
            n140 = call "Timeout.vi"("Start Time In"=w412, "Limit In"=w411) -> ("Timeout"=w410:bool)  [unwired: 8 in, 1 out]
            n141 = call <vilib>:"WPI_GyroReset.vi"("GyroDevRef"=w413) -> ("GyroDevRef"=w408:T9)  [unwired: 9 in, 1 out]
            n142 = call <vilib>:"WPI_RobotDriveTankDrive.vi"("Right axis value"=0.0, "Left axis value"=0.0, "RobotDriveDevRef"=w416) -> ("RobotDriveDevRef"=w409:T8)  [unwired: 6 in, 2 out]
          }
        }
        frame #1 {
          n143 = while {
            tunnel: w420 -> [w429]
            tunnel: w419 -> [w423]
            tunnel: [w424] -> w418
            tunnel: [w423] -> w417
            stop <- w425 stop-if-true
            n144 = call-poly <vilib>:"NT Read Value.vi"("Name"="Gyro Angle") -> ("Numeric"=w421:dbl)  [unwired: 9 in, 1 out]
            n145 = Equal?(x=w421, y=180.0) -> (x = y?=w425:bool)
            n146 = call <vilib>:"WPI_RobotDriveTankDrive.vi"("Right axis value"=-0.5, "Left axis value"=0.5, "RobotDriveDevRef"=w429) -> ("RobotDriveDevRef"=w424:T8)  [unwired: 6 in, 2 out]
          }
        }
        frame #2 {
          n147 = Tick Count (ms)() -> (millisecond timer value=w433:u32)
          n148 = while {
            tunnel: w431 -> [w442]
            tunnel: w430 -> [w439]
            tunnel: w433 -> [w438]
            tunnel: 200 -> [w437]
            tunnel: [w435] -> _
            tunnel: [w434] -> _
            stop <- w436 stop-if-true
            n149 = call "Timeout.vi"("Start Time In"=w438, "Limit In"=w437) -> ("Timeout"=w436:bool)  [unwired: 8 in, 1 out]
            n150 = call <vilib>:"WPI_GyroReset.vi"("GyroDevRef"=w439) -> ("GyroDevRef"=w434:T9)  [unwired: 9 in, 1 out]
            n151 = call <vilib>:"WPI_RobotDriveTankDrive.vi"("Right axis value"=0.0, "Left axis value"=0.0, "RobotDriveDevRef"=w442) -> ("RobotDriveDevRef"=w435:T8)  [unwired: 6 in, 2 out]
          }
        }
      }
    }
    frame "NegativeNinety" {
      n152 = flat-sequence {
        tunnel: w448 -> [w454]
        tunnel: w447 -> [w453]
        tunnel: [w450] -> w446
        tunnel: [w449] -> w445
        tunnel: w446 -> [w467]
        tunnel: w445 -> [w466]
        tunnel: [w465] -> w444
        tunnel: [w464] -> w443
        tunnel: w444 -> [w478]
        tunnel: w443 -> [w477]
        frame #0 {
          n153 = Tick Count (ms)() -> (millisecond timer value=w452:u32)
          n154 = while {
            tunnel: w454 -> [w463]
            tunnel: w453 -> [w460]
            tunnel: w452 -> [w459]
            tunnel: 200 -> [w458]
            tunnel: [w456] -> w450
            tunnel: [w455] -> w449
            stop <- w457 stop-if-true
            n155 = call "Timeout.vi"("Start Time In"=w459, "Limit In"=w458) -> ("Timeout"=w457:bool)  [unwired: 8 in, 1 out]
            n156 = call <vilib>:"WPI_GyroReset.vi"("GyroDevRef"=w460) -> ("GyroDevRef"=w455:T9)  [unwired: 9 in, 1 out]
            n157 = call <vilib>:"WPI_RobotDriveTankDrive.vi"("Right axis value"=0.0, "Left axis value"=0.0, "RobotDriveDevRef"=w463) -> ("RobotDriveDevRef"=w456:T8)  [unwired: 6 in, 2 out]
          }
        }
        frame #1 {
          n158 = while {
            tunnel: w467 -> [w476]
            tunnel: w466 -> [w470]
            tunnel: [w471] -> w465
            tunnel: [w470] -> w464
            stop <- w472 stop-if-true
            n159 = call-poly <vilib>:"NT Read Value.vi"("Name"="Gyro Angle") -> ("Numeric"=w469:dbl)  [unwired: 9 in, 1 out]
            n160 = Equal?(x=w469, y=-90.0) -> (x = y?=w472:bool)
            n161 = call <vilib>:"WPI_RobotDriveTankDrive.vi"("Right axis value"=0.5, "Left axis value"=-0.5, "RobotDriveDevRef"=w476) -> ("RobotDriveDevRef"=w471:T8)  [unwired: 6 in, 2 out]
          }
        }
        frame #2 {
          n162 = Tick Count (ms)() -> (millisecond timer value=w480:u32)
          n163 = while {
            tunnel: w478 -> [w489]
            tunnel: w477 -> [w486]
            tunnel: w480 -> [w485]
            tunnel: 200 -> [w484]
            tunnel: [w482] -> _
            tunnel: [w481] -> _
            stop <- w483 stop-if-true
            n164 = call "Timeout.vi"("Start Time In"=w485, "Limit In"=w484) -> ("Timeout"=w483:bool)  [unwired: 8 in, 1 out]
            n165 = call <vilib>:"WPI_GyroReset.vi"("GyroDevRef"=w486) -> ("GyroDevRef"=w481:T9)  [unwired: 9 in, 1 out]
            n166 = call <vilib>:"WPI_RobotDriveTankDrive.vi"("Right axis value"=0.0, "Left axis value"=0.0, "RobotDriveDevRef"=w489) -> ("RobotDriveDevRef"=w482:T8)  [unwired: 6 in, 2 out]
          }
        }
      }
    }
  }
